vi "Get Column Width.vi"(7 "Sheet Name":string, 8 "error in":errorcluster, 10 "Column":string="A", 11 "SpreadsheetDoc":refnum<k24>) -> (0 "error out":errorcluster, 2 "Width":dbl, 3 "SpreadsheetDoc out":refnum<k24>)   [LabVIEW 2019, in "Open Xml.lvlib"]
uses:
  Open Xml.lvlib
  D:/git/Open-Xml-LabVIEW/Source/DocumentFormat.OpenXml.dll
  DocumentFormat.OpenXml.dll
  D:/git/Open-Xml-LabVIEW/Source/DocumentFormat.OpenXml.Framework.dll
  DocumentFormat.OpenXml.Framework.dll
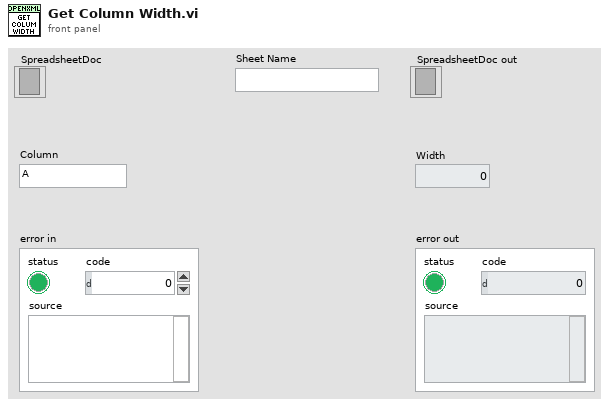
[diagram p1: front panel]
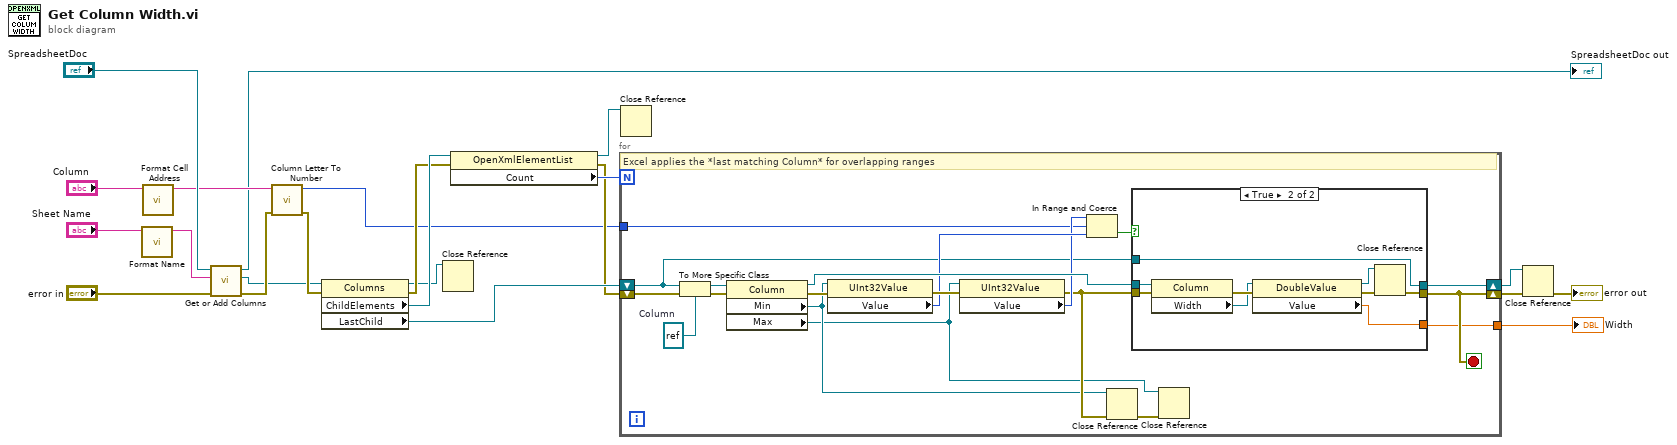
[diagram p0: block diagram]
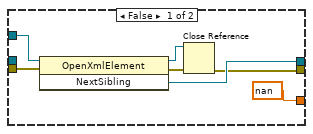
[diagram p2: hidden frame]
diagram:
  n1 = call "Format Name.vi"("Sheet Name"="Sheet Name") -> ("Formatted Sheet Name"=w19:string)  [unwired: 10 in]
  n2 = call "Format Cell Address.vi"("Cell Address"="Column") -> ("Formatted Cell Address"=w17:string)  [unwired: 10 in]
  n3 = call "Get or Add Columns.vi"("error in"="error in", "Sheet Name"=w19, "SpreadsheetDoc in"="SpreadsheetDoc") -> ("error out"=w16:errorcluster, "Columns"=w13:refnum<k24>, "SpreadsheetDoc out"=→"SpreadsheetDoc out":refnum<k24>)  [unwired: 6 in]
  n4 = call "Column Letter To Number.vi"("error in"=w16, "Letter"=w17) -> ("error out"=w15:errorcluster, "Number"=w5:i32)  [unwired: 8 in]
  n5 = property class="Columns"(reference=w13, error in=w15) -> (reference out=w1:refnum<k24>, error out=w9:errorcluster, "ChildElements"=w10:refnum<k24>, "LastChild"=w11:refnum<k24>)
  n6 = Close Reference(reference=w1) -> ()  [unwired: 1 in, 1 out]
  n7 = property class="OpenXmlElementList"(reference=w10, error in=w9) -> (reference out=w7:refnum<k24>, error out=w6:errorcluster, "Count"=w8:i32)
  n8 = for {
    N: w8 -> [_]
    shift-right: [w38] -> w12
    shift-left: w6 -> [w39]
    shift-right: [w37] -> w2
    shift-left: w11 -> [w27]
    tunnel: w5 -> [w30]
    tunnel: [w28] -> w4
    stop <- w38 stop-if-true
    w40 = refnum<k24> refnum  # Column
    # "Excel applies the *last matching Column* for overlapping ranges"
    n9 = To More Specific Class(target class=w40, reference=w27, error in=w39) -> (specific class reference=w36:refnum<k24>, error out=w41:errorcluster)
    n10 = property class="Column"(reference=w36, error in=w41) -> (reference out=w35:refnum<k24>, error out=w33:errorcluster, "Min"=w24:refnum<k24>, "Max"=w23:refnum<k24>)
    n11 = property class="UInt32Value"(reference=w24, error in=w33) -> (error out=w34:errorcluster, "Value"=w32:u32)  [unwired: 1 out]
    n12 = property class="UInt32Value"(reference=w23, error in=w34) -> (error out=w26:errorcluster, "Value"=w31:u32)  [unwired: 1 out]
    n13 = In Range and Coerce(upper limit=w31, x=w30, lower limit=w32) -> (In Range?=w29:bool)  [unwired: 1 out]
    n14 = Close Reference(reference=w24, error in (no error)=w26) -> (error out=w25:errorcluster)
    n15 = case shown="True" w29 {
      tunnel: [w45 w50] -> w38
      tunnel: [w48 w49] -> w37
      tunnel: w35 -> [_ w56]
      tunnel: w26 -> [w47 w57]
      tunnel: [nan w53] -> w28
      tunnel: w27 -> [w43 w49]
      frame False {
        n16 = invoke class="OpenXmlElement" method="NextSibling"(reference=w43, error in=w47) -> (reference out=w44:refnum<k24>, error out=w46:errorcluster, "NextSibling"=w48:refnum<k24>)  [unwired: 1 in]
        n17 = Close Reference(reference=w44, error in (no error)=w46) -> (error out=w45:errorcluster)
      }
      frame True {
        n18 = property class="Column"(reference=w56, error in=w57) -> (error out=w55:errorcluster, "Width"=w54:refnum<k24>)  [unwired: 1 out]
        n19 = property class="DoubleValue"(reference=w54, error in=w55) -> (reference out=w51:refnum<k24>, error out=w52:errorcluster, "Value"=w53:dbl)
        n20 = Close Reference(reference=w51, error in (no error)=w52) -> (error out=w50:errorcluster)
      }
    }
    n21 = Close Reference(reference=w23, error in (no error)=w25) -> ()  [unwired: 1 out]
  }
  "Width" <- w4
  n22 = Close Reference(reference=w7) -> ()  [unwired: 1 in, 1 out]
  n23 = Close Reference(reference=w2, error in (no error)=w12) -> (error out=→"error out":errorcluster)
